vi "Sequence with Asynchronous Acquisition (Express).vi"() -> ()   [LabVIEW 2011]
doc: "The Sequence with Asynchronous Acquisition (Express) VI acquires multiple images and displays them in an array of image controls. A sequence is appropriate for applications where you must perform processing on multiple images. Asynchronous acquisition is useful for processing while the acquisition is in progress without delaying the acquisition.\n\nAn image control displays the array of images on the front panel. To acquire synchronously, refer to the Sequence or Sequence (Express) VI in the IMAQdx folder."
uses:
  Instance           3 56Saved   Sequence with Asynchronous Acquisition (Express) .vi
panel:
  out "Image Array":T1[](array[plugin-control])
  in  "Stop":bool
  in  "Number of Images":i32=5
  # "Overview: Demonstrates how to acquire an asynchronous sequence of images and displays them in an array of image display controls.\nRequirements: Vision Acquisition Software\nInstructions: Run the VI"
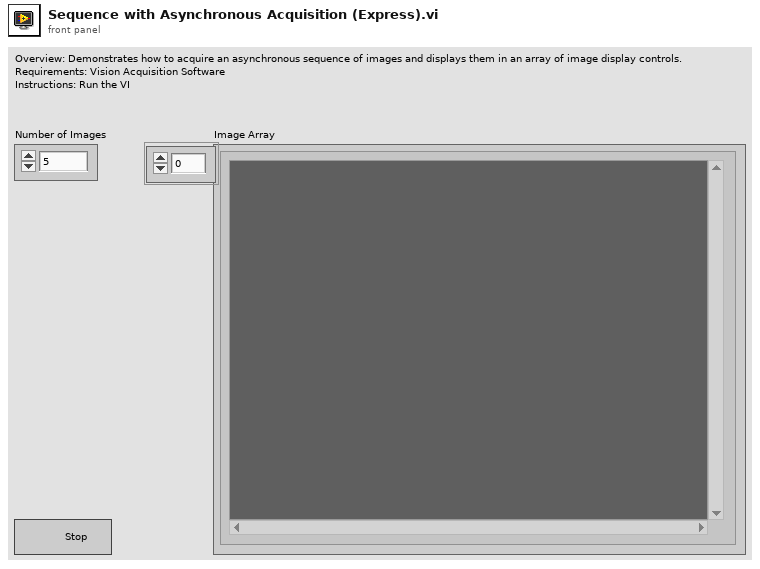
[diagram p1: front panel]
types:
  T1 = typedef "IMAQ Image.ctl" = refnum<image>
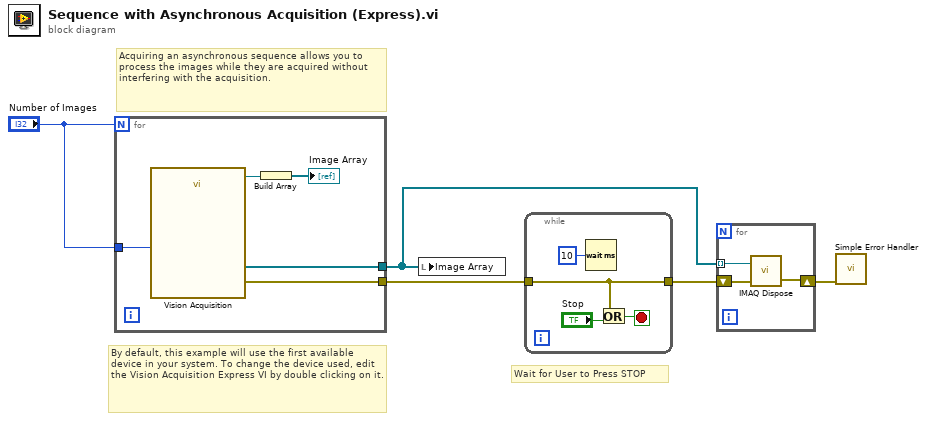
[diagram p0: block diagram]
diagram:
  # "Acquiring an asynchronous sequence allows you to process the images while they are acquired without interfering with the acquisition."
  # "Wait for User to Press STOP"
  # "By default, this example will use the first available device in your system. To change the device used, edit the Vision Acquisition Express VI by double clicking on it."
  n1 = for {
    N: "Number of Images" -> [_]
    tunnel: [w6] -> w1
    tunnel: [w9] -> w5
    tunnel: "Number of Images" -> [w7]
    n2 = call "Vision Acquisition"("Number of Images"=w7) -> ("Image Out"=w8:T1, "All Images Out"=w6:refnum<image>[], "error out"=w9:errorcluster)  [unwired: 1 in, 23 out]
    n3 = Build Array(w8) -> (→"Image Array":T1[])
  }
  n4 = local write "Image Array"(w1) -> ()
  n5 = while {
    tunnel: [w11] -> w4
    tunnel: w5 -> [w11]
    stop <- w12 stop-if-true
    n6 = Wait (ms)(milliseconds to wait=u32 10) -> ()  [unwired: 1 out]
    n7 = Or(x=w11, y="Stop") -> (x .or. y?=w12:bool)
  }
  n8 = for {
    tunnel: w1 -> [w17] mode=indexing
    shift-right: [w15] -> w3
    shift-left: w4 -> [w16]
    n9 = call "IMAQ Dispose"("Image"=w17, "error in (no error)"=w16) -> ("error out"=w15:errorcluster)  [unwired: 1 in, 3 out]
  }
  n10 = call <vilib>:"Simple Error Handler.vi"("error in (no error)"=w3) -> ()  [unwired: 1 in, 8 out]
